vi "PXI Scope.vi"() -> ()   [LabVIEW 2013]
uses:
  <instrlib>/niScope/Controls/niScope trigger source.ctl
  <instrlib>/niScope/Controls/niScope trigger coupling.ctl
  <instrlib>/niScope/Controls/niScope trigger slope.ctl
  <vilib>/Utility/miscctls.llb/LVPointTypeDef.ctl
  <instrlib>/niScope/Controls/niScope vertical coupling.ctl
  Database2.0/Public API/Signal.ctl
  Database2.0/Private/Role ID.ctl
  Database2.0/Private/Hardware ID.ctl
  <userlib>/_OpenG.lib/comparison/comparison.llb/DBL Changed__ogtk.vi
  <instrlib>/niScope/Configure/Trigger/niScope Configure Trigger Edge.vi
  <instrlib>/niScope/Configure/Trigger/niScope Configure Trigger Immediate.vi
  <instrlib>/niScope/Acquire/Fetch/niScope Multi Fetch Cluster.vi
panel:
  in  "Sampling rate":dbl=1000000.0 min=1000.0 max=1000000000.0 format="%#_2p"
  in  "min record length":i32=100000 min=1
  in  "trigger slope":T1=1 caption="trigger slope (Positive)"
  in  "trigger coupling":T2=1 caption="trigger coupling (DC)" items=["AC"=0, "DC"=1, "HF Reject"=3, "LF Reject"=4, "AC Plus HF Reject"=1001]
  in  "trigger source":T3="0" caption="trigger source (Channel 0)"
  out "Next Filename":string
  in  "File Name":string="test"
  in  "Save Path":path=path "G:/Local_Scope_Cache"
  in  "Write to Disk?":bool
  in  "Trigger Type":u16(ring) items=["Normal", "Automatic"]
  out "Avg. Rate":dbl format="%#.3g"
  in  "Ref. Pos.":dbl=40.0 format="%#_13g"
  in  "Reset Count":bool
  in  "Time (s)":dbl=0.1 min=1e-10 format="%.2p"
  in  "Clear Errors?":bool
  out "No. of Events":i32
  out "error out":errorcluster
  in  "stop":bool
  out "Scope":waveform(dbl)[](graph)
  in  "trigger level":dbl=0.5 format="%.4f"
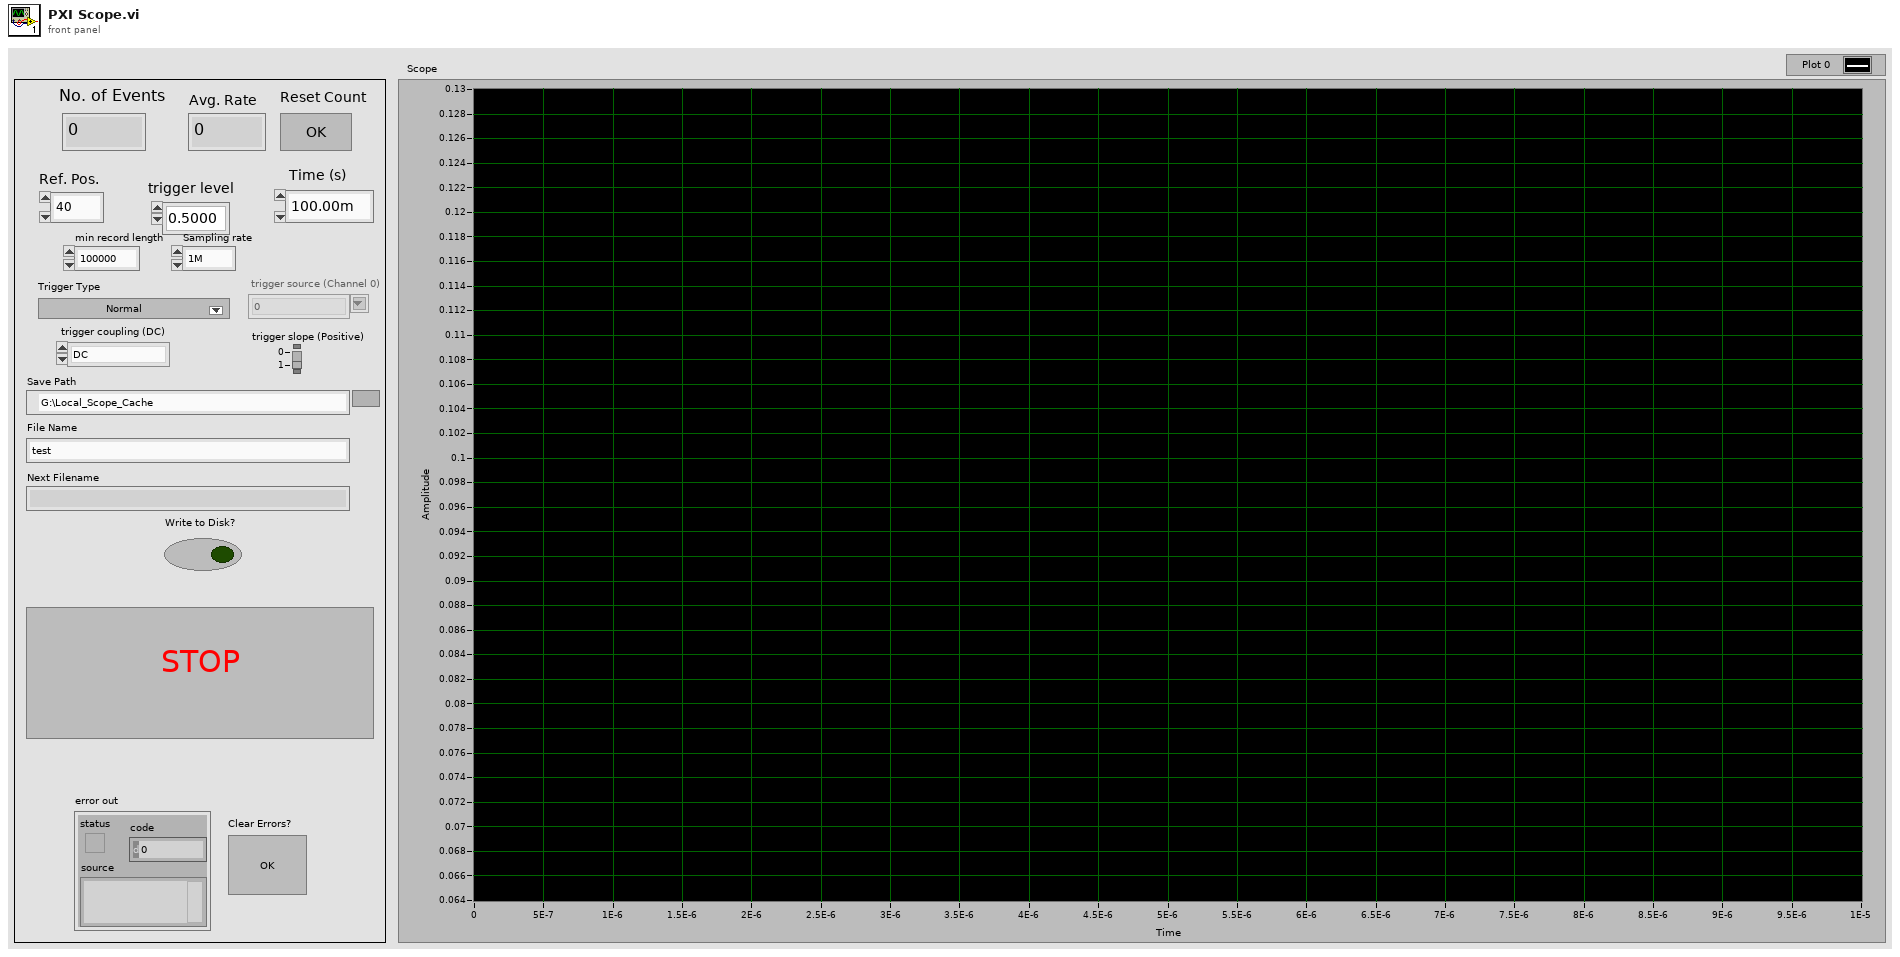
[diagram p1: front panel]
types:
  T1 = typedef "niScope trigger slope.ctl" = i32
  T2 = typedef "niScope trigger coupling.ctl" = u16
  T3 = typedef "niScope trigger source.ctl" = string
  T4 = typedef "LVPointTypeDef.ctl" = cluster{"Horizontal":i16, "Vertical":i16}
  T5 = enum8{"Enabled", "Disabled", "Disabled and Grayed Out"}
  T6 = cluster{"relativeInitialX":dbl, "xIncrement":dbl, "wfm":dbl[]}[]
  T7 = typedef "Hardware ID.ctl" = enum16{"Unknown", "CSA 1", "CSA 2", "CSA 3", "CSA 4", "CSA 5", "CSA 6"}
  T8 = typedef "Role ID.ctl" = enum16{"First_Detector", "Second_Detector", "Third_Detector", "LeCroy_CH1", "LeCroy_CH2", "LeCroy_CH3", "LeCroy_CH4", "PSU"}
  T9 = typedef "niScope vertical coupling.ctl" = i32
  T10 = typedef "Signal.ctl" = cluster{"Signal ID":i64, "Time Stamp":timestamp, "Dust Event ID":i64, "Role ID":T8, "Data":sgl[], "Signal Length":i32, "dt":sgl, "Offset":dbl, "Hardware ID":T7}
  T11 = cluster{"relativeInitialX":dbl, "xIncrement":dbl, "wfm":dbl[]}
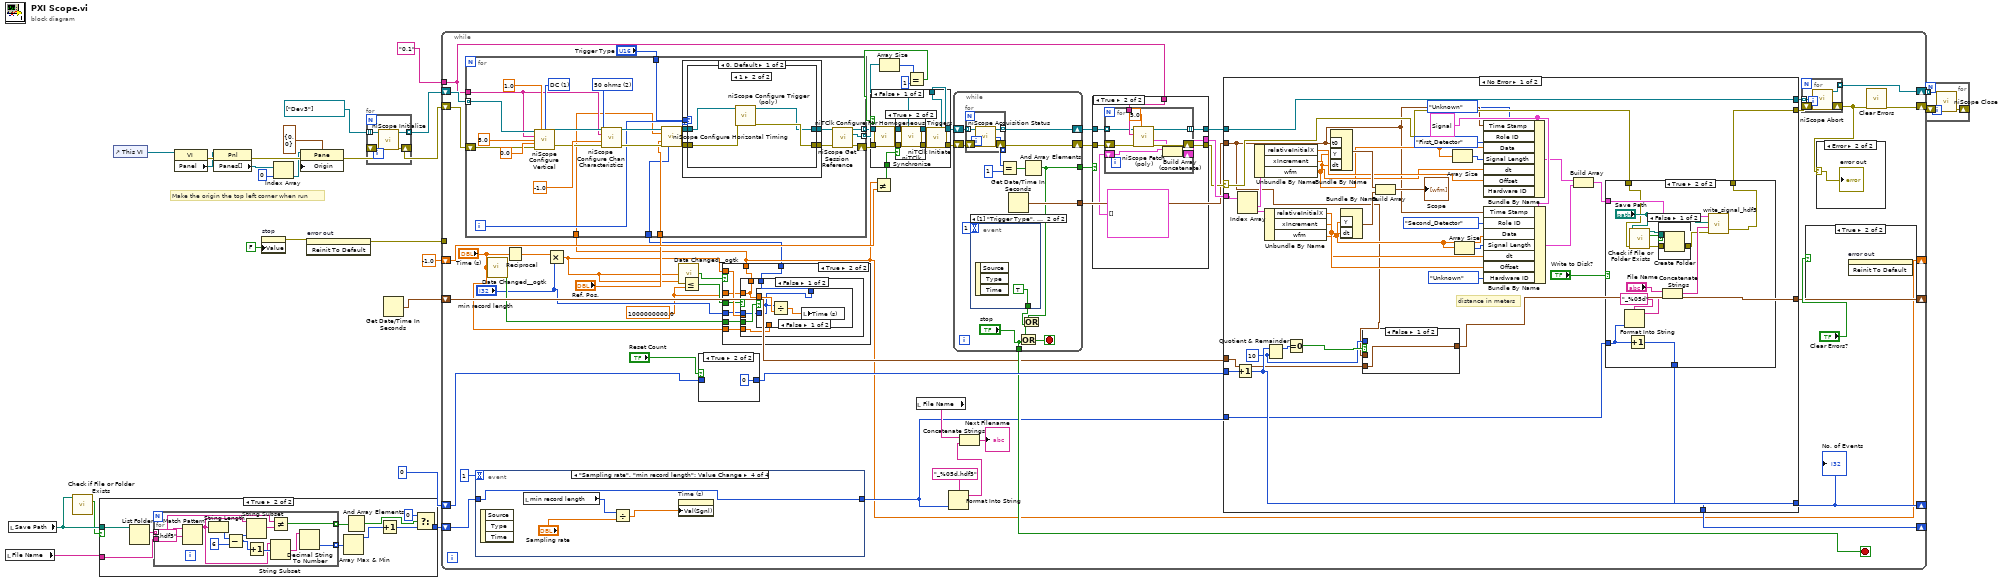
[diagram p0: block diagram]
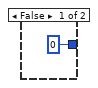
[diagram p2: hidden frame]
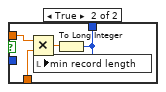
[diagram p4: hidden frame]
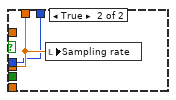
[diagram p5: hidden frame]
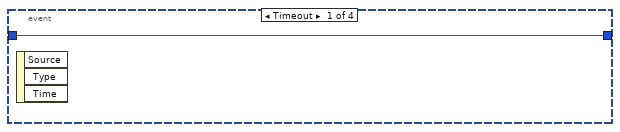
[diagram p6: hidden frame]
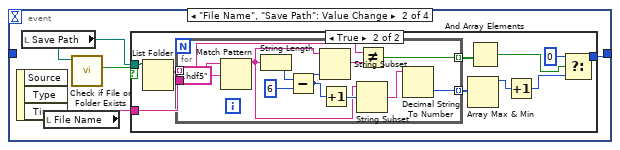
[diagram p7: hidden frame]
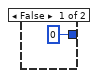
[diagram p8: hidden frame]
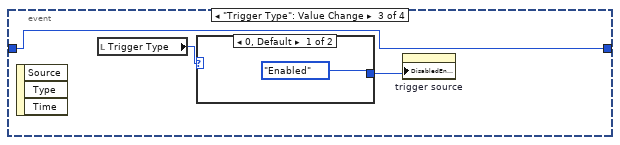
[diagram p9: hidden frame]
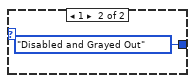
[diagram p10: hidden frame]
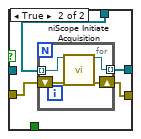
[diagram p12: hidden frame]
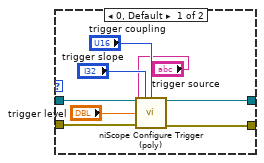
[diagram p14: hidden frame]
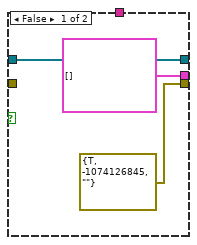
[diagram p16: hidden frame]
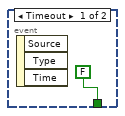
[diagram p17: hidden frame]
diagram:
  # "Make the origin the top left corner when run"
  n1 = local read "File Name"() -> (w4:string)
  n2 = local read "Save Path"() -> (w2:path)
  n3 = call <vilib>:"Check if File or Folder Exists.vi"("path"=w2) -> ("file or folder exists?"=w1:bool)  [unwired: 8 in, 2 out]
  n4 = case shown="True" w1 {
    tunnel: w4 -> [_ w36]
    tunnel: [0 ("t") w31] -> w3
    tunnel: w2 -> [_ w28]
    frame False {
    }
    frame True {
      n5 = List Folder(path=w28) -> (filenames=w32:string[])  [unwired: 3 in, 3 out]
      n6 = for {
        tunnel: w32 -> [w47] mode=indexing
        tunnel: w36 -> [w39]
        tunnel: [w48] -> w35 mode=indexing
        tunnel: [w38] -> w27 mode=indexing
        n7 = Match Pattern(string=w47, regular expression=".hdf5") -> (before substring=w37:string)  [unwired: 1 in, 3 out]
        n8 = String Length(string=w37) -> (length=w45:i32)
        n9 = Subtract(x=w45, y=6) -> (x-y=w43:i32)
        n10 = String Subset(string=w37, length (rest)=w43) -> (substring=w40:string)  [unwired: 1 in]
        n11 = Increment(x=w43) -> (x+1=w42:i32)
        n12 = String Subset(string=w37, offset (0)=w42) -> (substring=w41:string)  [unwired: 1 in]
        n13 = Not Equal?(x=w39, y=w40) -> (x != y?=w38:bool)
        n14 = Decimal String To Number(string=w41) -> (number=w48:i32)  [unwired: 2 in, 1 out]
      }
      n15 = Array Max & Min(array=w35) -> (max value=w34:i32)  [unwired: 3 out]
      n16 = And Array Elements(Boolean array=w27) -> (logical AND=w29:bool)
      n17 = Increment(x=w34) -> (x+1=w33:i32)
      n18 = Select(t=0, s=w29, f=w33) -> (s? t:f=w31:i32)
    }
  }
  n19 = control-ref of="This VI"() -> (w17:refnum<vi>)
  n20 = property class="VI"(reference=w17) -> (error out=w24:errorcluster, "Panel"=w18:refnum<vi>)  [unwired: 1 in, 1 out]
  n21 = property class="Pnl"(reference=w18, error in=w24) -> (error out=w23:errorcluster, "Panes[]"=w22:refnum<vi>[])  [unwired: 1 out]
  n22 = property on="stop" class="Bool (strict)"("Value"=FALSE ("stop")) -> (error out=w7:errorcluster)  [unwired: 2 in, 1 out]
  n23 = Index Array(array=w22, index=0) -> (element=w20:refnum<vi>)
  n24 = property class="Pane"(reference=w20, error in=w23, "Origin"=T4 {"Horizontal"=0, "Vertical"=0}) -> (error out=w25:errorcluster)  [unwired: 1 out]
  n25 = invoke on="error out" class="Clust (strict)" method="Reinit To Default"(error in=w7) -> (error out=w14:errorcluster)  [unwired: 2 in, 2 out]
  n26 = for {
    tunnel: [w50] -> w13 mode=indexing
    tunnel: refnum<k15>[] ["Dev3"] -> [w49] mode=indexing
    shift-right: [w51] -> w9
    shift-left: w25 -> [w52]
    n27 = call <instrlib>:"niScope Initialize.vi"("resource name"=w49, "error in"=w52) -> ("instrument handle"=w50:refnum<k15>, "error out"=w51:errorcluster)  [unwired: 12 in]
  }
  n28 = Get Date/Time In Seconds() -> (seconds since 1Jan1904=w6:timestamp)
  n29 = while {
    tunnel: "0,1" ("channels") -> [w103]
    shift-right: [w89] -> w12
    shift-left: w13 -> [w104]
    shift-right: [w88] -> w11
    shift-left: w9 -> [w105]
    shift-right: [w98] -> _
    shift-left: 0 -> [w87]
    tunnel: w14 -> [_]
    shift-right: [w60] -> _
    shift-left: -1.0 ("min sample rate") -> [w84]
    shift-right: [w78] -> _
    shift-left: w6 -> [w79]
    shift-right: [w70] -> _
    shift-left: w3 -> [w69]
    stop <- w80 stop-if-true
    w53 = 1000000000.0 ("y")
    n30 = event shown="[3] \"Sampling rate\", \"min record length\": Value Change" {
      selector: _ -> [_ _ _ _]
      dyn-events: _ -> [_ _ _ _]
      timeout: 1 -> [_ _ _ _]
      tunnel: w69 -> [w130 _ w158 w163]
      tunnel: [w130 w134 w158 w163] -> w64
      event Timeout {
        n31 = event-data() -> ()  [unwired: 1 in, 3 out]
      }
      event "File Name", "Save Path": Value Change {
        n32 = event-data() -> ()  [unwired: 1 in, 3 out]
        n33 = local read "Save Path"() -> (w132:path)
        n34 = local read "File Name"() -> (w133:string)
        n35 = call <vilib>:"Check if File or Folder Exists.vi"("path"=w132) -> ("file or folder exists?"=w131:bool)  [unwired: 8 in, 2 out]
        n36 = case shown="True" w131 {
          tunnel: [0 ("t") w145] -> w134
          tunnel: w132 -> [_ w142]
          tunnel: w133 -> [_ w138]
          frame False {
          }
          frame True {
            n37 = List Folder(path=w142) -> (filenames=w139:string[])  [unwired: 3 in, 3 out]
            n38 = for {
              tunnel: w139 -> [w156] mode=indexing
              tunnel: w138 -> [w148]
              tunnel: [w157] -> w137 mode=indexing
              tunnel: [w147] -> w136 mode=indexing
              n39 = Match Pattern(string=w156, regular expression=".hdf5") -> (before substring=w146:string)  [unwired: 1 in, 3 out]
              n40 = String Length(string=w146) -> (length=w154:i32)
              n41 = Subtract(x=w154, y=6) -> (x-y=w152:i32)
              n42 = String Subset(string=w146, length (rest)=w152) -> (substring=w149:string)  [unwired: 1 in]
              n43 = Increment(x=w152) -> (x+1=w151:i32)
              n44 = String Subset(string=w146, offset (0)=w151) -> (substring=w150:string)  [unwired: 1 in]
              n45 = Not Equal?(x=w148, y=w149) -> (x != y?=w147:bool)
              n46 = Decimal String To Number(string=w150) -> (number=w157:i32)  [unwired: 2 in, 1 out]
            }
            n47 = Array Max & Min(array=w137) -> (max value=w140:i32)  [unwired: 3 out]
            n48 = And Array Elements(Boolean array=w136) -> (logical AND=w141:bool)
            n49 = Increment(x=w140) -> (x+1=w144:i32)
            n50 = Select(t=0, s=w141, f=w144) -> (s? t:f=w145:i32)
          }
        }
      }
      event "Trigger Type": Value Change {
        n51 = event-data() -> ()  [unwired: 1 in, 3 out]
        n52 = local read "Trigger Type"() -> (w160:u16)
        n53 = case shown="0, Default" w160 {
          tunnel: [T5."Enabled" ("Disabled") T5."Disabled and Grayed Out" ("Disabled")] -> w159
          frame 0, Default {
          }
          frame 1 {
          }
        }
        n54 = property on="trigger source" class="CmbBox (strict)"("DisabledEnum"=w159) -> ()  [unwired: 2 in, 2 out]
      }
      event "Sampling rate", "min record length": Value Change {
        n55 = event-data() -> ()  [unwired: 1 in, 3 out]
        n56 = local read "min record length"() -> (w166:i32)
        n57 = Divide(x=w166, y="Sampling rate") -> (x/y=w164:dbl)
        n58 = property on="Time (s)" class="DigNum (strict)"("Val(Sgnl)"=w164) -> ()  [unwired: 2 in, 2 out]
      }
    }
    n59 = call-poly <userlib>:"Data Changed__ogtk.vi"("DBL"="Time (s)") -> ("Changed"=w57:bool)
    n60 = Reciprocal(x="Time (s)") -> (1/x=w62:dbl)
    n61 = Multiply(x=w62, y="min record length") -> (x*y=w61:dbl)
    n62 = call-poly <userlib>:"Data Changed__ogtk.vi"("DBL"=w61) -> ("Changed"=w59:bool)
    n63 = Less Or Equal?(x=w61, y=w53) -> (x <= y?=w58:bool)
    n64 = case shown="True" "Reset Count" {
      tunnel: w87 -> [w190 _]
      tunnel: [w190 0] -> w86
      frame False {
      }
      frame True {
      }
    }
    n65 = case shown="True" w59 {
      tunnel: w61 -> [w107 w115]
      tunnel: [w107 w113] -> w60
      tunnel: w58 -> [_ w114]
      tunnel: w57 -> [_ w112]
      tunnel: "min record length" -> [w106 w111]
      tunnel: [w106 w110] -> w55
      tunnel: "Time (s)" -> [_ w109]
      tunnel: w53 -> [_ w108]
      frame False {
      }
      frame True {
        n66 = case shown="False" w114 {
          tunnel: w115 -> [_ w129]
          tunnel: [w117 w129] -> w113
          tunnel: w112 -> [w120 _]
          tunnel: w111 -> [w118 w128]
          tunnel: [w116 w128] -> w110
          tunnel: w109 -> [w119 _]
          tunnel: w108 -> [w117 _]
          frame False {
            n67 = case shown="False" w120 {
              tunnel: w119 -> [_ w126]
              tunnel: w118 -> [w121 _]
              tunnel: w117 -> [w123 w127]
              tunnel: [w121 w124] -> w116
              frame False {
                n68 = Divide(x=w121, y=w123) -> (x/y=w122:dbl)
                n69 = local write "Time (s)"(w122) -> ()
              }
              frame True {
                n70 = Multiply(x=w127, y=w126) -> (x*y=w125:dbl)
                n71 = To Long Integer(number=w125) -> (32bit integer=w124:i32)
                n72 = local write "min record length"(w124) -> ()
              }
            }
          }
          frame True {
            n73 = local write "Sampling rate"(w129) -> ()
          }
        }
      }
    }
    n74 = for {
      tunnel: w104 -> [w215] mode=indexing
      tunnel: [w203] -> w72 mode=indexing
      tunnel: w103 -> [w205]
      shift-right: [w201] -> w91
      shift-left: w105 -> [w216]
      tunnel: [w200] -> w92 mode=indexing
      tunnel: w60 -> [w199]
      tunnel: "Ref. Pos." -> [w198]
      tunnel: "Trigger Type" -> [w197]
      tunnel: w55 -> [w196]
      i -> [w204]
      w214 = u32 2 items=["1 mega ohm"=0, "50 ohms"=2] ("input impedance")
      w217 = T9 1 items=["AC", "DC", "Ground"] ("vertical coupling")
      n75 = call <instrlib>:"niScope Configure Vertical.vi"("instrument handle"=w215, "probe attenuation"=1.0, "vertical coupling"=w217, "channels"=w205, "vertical range"=5.0, "vertical offset"=0.0, "error in"=w216) -> ("instrument handle out"=w211:refnum<k15>, "error out"=w212:errorcluster)  [unwired: 7 in]
      n76 = call <instrlib>:"niScope Configure Chan Characteristics.vi"("instrument handle"=w211, "channels"=w205, "input impedance"=w214, "maximum input frequency"=-1.0, "error in"=w212) -> ("instrument handle out"=w209:refnum<k15>, "error out"=w210:errorcluster)  [unwired: 9 in]
      n77 = call <instrlib>:"niScope Configure Horizontal Timing.vi"("instrument handle"=w209, "min sample rate"=w199, "reference position"=w198, "error in"=w210, "min record length"=w196) -> ("instrument handle out"=w208:refnum<k15>, "error out"=w207:errorcluster)  [unwired: 9 in]
      n78 = case shown="0, Default" w204 {
        tunnel: w208 -> [w225 w239]
        tunnel: w207 -> [w224 w238]
        tunnel: [w223 w239] -> w206
        tunnel: [w222 w238] -> w202
        tunnel: w197 -> [w221 _]
        frame 0, Default {
          n79 = case shown="1" w221 {
            tunnel: w225 -> [w233 w237]
            tunnel: w224 -> [w232 w236]
            tunnel: [w228 w234] -> w223
            tunnel: [w227 w235] -> w222
            frame 0, Default {
              n80 = call-poly <instrlib>:"niScope Configure Trigger (poly).vi"("instrument handle"=w233, "trigger slope"="trigger slope", "trigger coupling"="trigger coupling", "trigger source"="trigger source", "trigger level"="trigger level", "error in"=w232) -> ("instrument handle out"=w228:refnum<k15>, "error out"=w227:errorcluster)  [unwired: 8 in]
            }
            frame 1 {
              n81 = call-poly <instrlib>:"niScope Configure Trigger (poly).vi"("instrument handle"=w237, "error in"=w236) -> ("instrument handle out"=w234:refnum<k15>, "error out"=w235:errorcluster)  [unwired: 12 in]
            }
          }
        }
        frame 1 {
        }
      }
      n82 = call <instrlib>:"niScope Get Session Reference.vi"("instrument handle"=w206, "error in"=w202) -> ("instrument handle out"=w203:refnum<k15>, "session reference"=w200:refnum<k20>, "error out"=w201:errorcluster)  [unwired: 11 in]
    }
    n83 = Not Equal?(x=w60, y=w84) -> (x != y?=w83:bool)
    n84 = Array Size(array=w72) -> (size(s)=w75:i32)
    n85 = Equal?(x=w75, y=1) -> (x = y?=w73:bool)
    n86 = case shown="False" w73 {
      tunnel: w92 -> [w175 _]
      tunnel: w91 -> [w174 w184]
      tunnel: [w169 w183] -> w90
      tunnel: w83 -> [w168 _]
      tunnel: w72 -> [w167 w185]
      tunnel: [w167 w182] -> w71
      frame False {
        n87 = call <instrlib>:"niTClk Configure For Homogeneous Triggers.vi"("error in (no error)"=w174, "sessions"=w175) -> ("error out"=w172:errorcluster, "sessions out"=w173:refnum<k20>[])  [unwired: 8 in]
        n88 = case shown="True" w168 {
          tunnel: w173 -> [w177 w181]
          tunnel: w172 -> [w176 w180]
          tunnel: [w177 w179] -> w171
          tunnel: [w176 w178] -> w170
          frame False {
          }
          frame True {
            n89 = call <instrlib>:"niTClk Synchronize.vi"("error in (no error)"=w180, "sessions"=w181) -> ("error out"=w178:errorcluster, "sessions out"=w179:refnum<k20>[])  [unwired: 8 in]
          }
        }
        n90 = call <instrlib>:"niTClk Initiate.vi"("error in (no error)"=w170, "sessions"=w171) -> ("error out"=w169:errorcluster)  [unwired: 8 in, 1 out]
      }
      frame True {
        n91 = for {
          tunnel: w185 -> [w189] mode=indexing
          tunnel: [w186] -> w182 mode=indexing
          shift-right: [w187] -> w183
          shift-left: w184 -> [w188]
          n92 = call <instrlib>:"niScope Initiate Acquisition.vi"("instrument handle"=w189, "error in"=w188) -> ("instrument handle out"=w186:refnum<k15>, "error out"=w187:errorcluster)  [unwired: 12 in]
        }
      }
    }
    n93 = local read "File Name"() -> (w65:string)
    n94 = Format Into String(format string="_%05d.hdf5", w64) -> (resulting string=w66:string)  [unwired: 2 in, 1 out]
    n95 = while {
      shift-right: [w269] -> w95
      shift-left: w71 -> [w272]
      shift-right: [w270] -> w94
      shift-left: w90 -> [w271]
      tunnel: [w261] -> w93
      tunnel: [w262] -> w82
      tunnel: ["stop"] -> w80
      stop <- w260 stop-if-true
      n96 = for {
        tunnel: w272 -> [w277] mode=indexing
        tunnel: [w274] -> w269 mode=indexing
        tunnel: [w273] -> w268 mode=indexing
        shift-right: [w275] -> w270
        shift-left: w271 -> [w276]
        n97 = call <instrlib>:"niScope Acquisition Status.vi"("instrument handle"=w277, "error in"=w276) -> ("instrument handle out"=w274:refnum<k15>, "acquisition status"=w273:i32, "error out"=w275:errorcluster)  [unwired: 11 in]
      }
      n98 = event shown="[1] \"Trigger Type\", \"Clear Errors?\", \"Time (s)\", \"Reset Count\", \"Ref. Pos.\", \"File Name\", \"Save Path\", \"trigger source\", \"trigger coupling\", \"trigger slope\", \"min record length\", \"Sampling rate\": Value Change" {
        selector: _ -> [_ _]
        dyn-events: _ -> [_ _]
        timeout: 1 -> [_ _]
        tunnel: [FALSE TRUE] -> w265
        event Timeout {
          n99 = event-data() -> ()  [unwired: 1 in, 3 out]
        }
        event "Trigger Type", "Clear Errors?", "Time (s)", "Reset Count", "Ref. Pos.", "File Name", "Save Path", "min record length", "Sampling rate": Value Change {
          n100 = event-data() -> ()  [unwired: 1 in, 3 out]
        }
      }
      n101 = Equal?(x=w268, y=1) -> (x = y?=w263:bool[])
      n102 = Get Date/Time In Seconds() -> (seconds since 1Jan1904=w262:timestamp)
      n103 = And Array Elements(Boolean array=w263) -> (logical AND=w261:bool)
      n104 = Or(x=w261, y=w265) -> (x .or. y?=w264:bool)
      n105 = Or(x=w264, y="stop") -> (x .or. y?=w260:bool)
    }
    n106 = Concatenate Strings(w65, w66) -> (→"Next Filename":string)
    n107 = case shown="True" w93 {
      tunnel: w103 -> [_ w249]
      tunnel: [T6 [] ("waveform") w243] -> w102
      tunnel: [w242 w248] -> w101
      tunnel: [errorcluster {"status"=TRUE, "code"=-1074126845, "source"=""} ("error out") w247] -> w99
      tunnel: w95 -> [w242 w246]
      tunnel: w94 -> [_ w245]
      frame False {
      }
      frame True {
        n108 = for {
          tunnel: w249 -> [w258]
          tunnel: [w256] -> w248 mode=indexing
          tunnel: w246 -> [w254] mode=indexing
          shift-right: [w251] -> w243
          shift-left: T6 [] ("waveform") -> [w250]
          shift-right: [w255] -> w247
          shift-left: w245 -> [w253]
          n109 = call-poly <instrlib>:"niScope Fetch (poly).vi"("timeout"=5.0, "error in"=w253, "channels"=w258, "instrument handle"=w254) -> ("error out"=w255:errorcluster, "waveform"=w252:T6, "instrument handle out"=w256:refnum<k15>)  [unwired: 4 in, 1 out]
          n110 = Build Array (concatenate)(w250, w252) -> (w251:T6)
        }
      }
    }
    n111 = case shown="No Error" w99 {
      selector: w99 -> [w302 w348]
      tunnel: w102 -> [w311 _]
      tunnel: w101 -> [w310 w351]
      tunnel: [w310 w351] -> w100
      tunnel: w86 -> [w283 w346]
      tunnel: [w309 w346] -> w98
      tunnel: [w301 w345] -> w97
      tunnel: w82 -> [w286 _]
      tunnel: w79 -> [w306 w344]
      tunnel: [w304 w344] -> w78
      tunnel: w64 -> [w282 w343]
      tunnel: [w281 w343] -> w70
      frame No Error {
        w300 = T10 {"Signal ID"=0, "Time Stamp"=timestamp(0 s since 1904-01-01), "Dust Event ID"=0, "Role ID"=enum."First_Detector", "Data"=[], "Signal Length"=0, "dt"=0.0, "Offset"=0.0, "Hardware ID"=enum."CSA 1"} ("Signal")
        w305 = 10 ("y")
        # "distance in meters"
        n112 = Increment(x=w283) -> (x+1=w309:i32)
        n113 = Index Array(array=w311) -> (element #1=w316:T11, element #2=w315:T11)  [unwired: 2 in]
        n114 = Unbundle By Name(w316) -> ("relativeInitialX"=w296:dbl, "xIncrement"=w295:dbl, "wfm"=w292:dbl[])
        n115 = Unbundle By Name(w315) -> ("relativeInitialX"=w294:dbl, "xIncrement"=w293:dbl, "wfm"=w290:dbl[])
        n116 = Quotient & Remainder(x=w309, y=w305) -> (x-y*floor(x/y)=w308:i32)  [unwired: 1 out]
        n117 = Equal To 0?(x=w308) -> (x = 0?=w307:bool)
        n118 = Bundle By Name("t0"=w286, "Y"=w292, "dt"=w295) -> (w314:waveform(dbl))  [unwired: 1 in]
        n119 = Bundle By Name("Y"=w290, "dt"=w293) -> (w313:waveform(dbl))  [unwired: 1 in]
        n120 = case shown="False" w307 {
          tunnel: w306 -> [w337 w342]
          tunnel: w286 -> [_ w338]
          tunnel: w305 -> [_ w340]
          tunnel: [w337 w338] -> w304
          frame False {
          }
          frame True {
            n121 = Subtract(x=w338, y=w342) -> (x-y=w341:dbl)
            n122 = Divide(x=w340, y=w341) -> (x/y=→"Avg. Rate":dbl)
          }
        }
        n123 = Build Array(w314, w313) -> (→"Scope":waveform(dbl)[])
        n124 = Array Size(array=w292) -> (size(s)=w291:i32)
        n125 = Array Size(array=w290) -> (size(s)=w289:i32)
        n126 = Bundle By Name(cluster=w300, "Time Stamp"=w286, "Role ID"=Role_ID."First_Detector", "Data"=w292, "Signal Length"=w291, "dt"=w295, "Offset"=w296, "Hardware ID"=Hardware_ID."Unknown") -> (w299:T10)
        n127 = Bundle By Name(cluster=w300, "Time Stamp"=w286, "Role ID"=Role_ID."Second_Detector", "Data"=w290, "Signal Length"=w289, "dt"=w293, "Offset"=w294, "Hardware ID"=Hardware_ID."Unknown") -> (w298:T10)
        n128 = Build Array(w299, w298) -> (w297:T10[])
        n129 = case shown="True" "Write to Disk?" {
          tunnel: w302 -> [w318 w324]
          tunnel: [w318 w319] -> w301
          tunnel: w297 -> [_ w332]
          tunnel: w282 -> [w317 w327]
          tunnel: [w317 w326] -> w281
          frame False {
          }
          frame True {
            n130 = Format Into String(format string="_%05d", w327) -> (resulting string=w329:string)  [unwired: 2 in, 1 out]
            n131 = Increment(x=w327) -> (x+1=w326:i32)
            n132 = call <vilib>:"Check if File or Folder Exists.vi"("error in (no error)"=w324, "path"="Save Path") -> ("error out"=w321:errorcluster, "file or folder exists?"=w323:bool, "dup path"=w320:path)  [unwired: 7 in]
            n133 = case shown="False" w323 {
              tunnel: w321 -> [w333 w336]
              tunnel: [w334 w336] -> w322
              tunnel: w320 -> [w335 _]
              frame False {
                n134 = Create Folder(path (use dialog)=w335, error in=w333) -> (error out=w334:errorcluster)  [unwired: 1 in, 2 out]
              }
              frame True {
              }
            }
            n135 = Concatenate Strings("File Name", w329) -> (w328:string)
            n136 = call "write_signal_hdf5.vi"("error in"=w322, "File Name"=w328, "Save Path"="Save Path", "Signal array"=w332) -> ("error out"=w319:errorcluster)  [unwired: 6 in, 1 out]
          }
        }
      }
      frame Error {
        n137 = Unbundle By Name(w348) -> ("code"=w350:i32)
        n138 = Equal?(x=w350, y=-1074126845) -> (x = y?=w347:bool)
        n139 = case shown="True" w347 {
          tunnel: [w352 w354] -> w345
          tunnel: w348 -> [w352 w353]
          frame False {
          }
          frame True {
            n140 = call <vilib>:"Clear Errors.vi"("error in (no error)"=w353) -> ("error out"=w354:errorcluster)  [unwired: 6 in]
          }
        }
      }
    }
    "No. of Events" <- w98
    n141 = for {
      tunnel: w100 -> [w195] mode=indexing
      shift-right: [w194] -> w77
      shift-left: w97 -> [w193]
      tunnel: [w192] -> w89 mode=indexing
      n142 = call <instrlib>:"niScope Abort.vi"("instrument handle"=w195, "error in"=w193) -> ("instrument handle out"=w192:refnum<k15>, "error out"=w194:errorcluster)  [unwired: 12 in]
    }
    n143 = case shown="True" "Clear Errors?" {
      frame False {
      }
      frame True {
        n144 = invoke on="error out" class="Clust (strict)" method="Reinit To Default"() -> ()  [unwired: 3 in, 3 out]
      }
    }
    n145 = case shown="Error" w77 {
      selector: w77 -> [_ w280]
      frame No Error {
      }
      frame Error {
        "error out" <- w280
      }
    }
    n146 = call <vilib>:"Clear Errors.vi"("error in (no error)"=w77) -> ("error out"=w88:errorcluster)  [unwired: 6 in]
  }
  n147 = for {
    tunnel: w12 -> [w357] mode=indexing
    shift-right: [w355] -> _
    shift-left: w11 -> [w356]
    n148 = call <instrlib>:"niScope Close.vi"("instrument handle"=w357, "error in"=w356) -> ("error out"=w355:errorcluster)  [unwired: 13 in]
  }
